vi "RotateDegrees.vi"() -> ()   [LabVIEW 2016]
uses:
  Refname/Motors.ctl
  Refname/Refname to String (Motors).vi
  <vilib>/addons/control/pid/pid.llb/PID (DBL).vi
  <vilib>/addons/control/pid/NI_PID_pid.lvlib
panel:
  in  "Threshold Wheel":dbl format="%#_13g"
  in  "PID Gains Wheel":T1={"proportional gain (Kc)"=1.0, "integral time (Ti, min)"=0.01, "derivative time (Td, min)"=0.0} {"derivative time (Td, min)" format="%.3f"; "integral time (Ti, min)" format="%.3f"; "proportional gain (Kc)" format="%.3f"}
  in  "Threshhold":dbl
  in  "PID gains Swerve":T1={"proportional gain (Kc)"=1.0, "integral time (Ti, min)"=0.01, "derivative time (Td, min)"=0.0} {"derivative time (Td, min)" format="%.3f"; "integral time (Ti, min)" format="%.3f"; "proportional gain (Kc)" format="%.3f"}
  in  "Radians to Turn":dbl format="%#_13g"
  in  "Encoder Position":dbl=22.222 format="%#_13g"
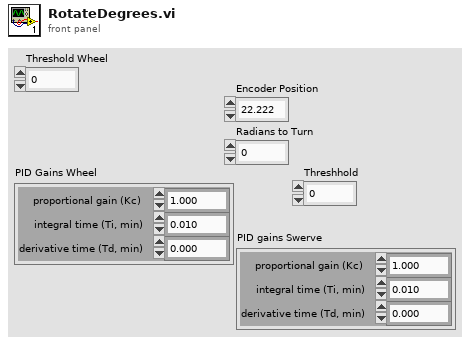
[diagram p1: front panel]
types:
  T1 = cluster{"proportional gain (Kc)":dbl, "integral time (Ti, min)":dbl, "derivative time (Td, min)":dbl}
  T2 = typedef "Motors.ctl" = enum16{"Wheel 1", "Swerve 1", "Wheel 2", "Swerve 2", "Wheel 3", "Swerve 3", "Wheel 4", "Swerve 4"}
  T3 = typedef "WPI_MotorControlDeviceRef.ctl" = cluster{"DeviceStatus":errorcluster, "Type":T4, "PWM":cluster{"PWM Channel":T5, "DeadBand":T6}, "CAN":cluster{"Device Number":u8, "SetOutput VI Ref":variant, "GetOutput VI Ref":variant, "Enable VI Ref":variant, "Disable VI Ref":variant, "Data":variant}, "Invert":bool}
  T4 = typedef "WPI_MotorControlType.ctl" = enum16{"PWM", "CAN"}
  T5 = typedef "FPGA_DIOPWMChannel.ctl" = enum8{"PWM 0", "PWM 1", "PWM 2", "PWM 3", "PWM 4", "PWM 5", "PWM 6", "PWM 7", "PWM 8", "PWM 9", "PWM MXP 0", "PWM MXP 1", "PWM MXP 2", "PWM MXP 3", "PWM MXP 4", "PWM MXP 5", "PWM MXP 6", "PWM MXP 7", "PWM MXP 8", "PWM MXP 9", "Invalid"}
  T6 = typedef "WPI_PWMDeadband.ctl" = cluster{"Name":string, "maxPositivePwm":i32, "minPositivePwm":i32, "centerPwm":i32, "maxNegativePwm":i32, "minNegativePwm":i32, "angularRange":u16}
  T7 = typedef "WPI_CANTalonSRX_GlobalStatus.ctl" = cluster{"Applied Throttle":dbl, "Module Enabled":bool, "CAN Error":errorcluster, "Closed Loop Error":dbl, "Forward Limit Switch Closed":bool, "Reverse Limit Switch Closed":bool, "Sensor Position":dbl, "Sensor Velocity":dbl, "Current":dbl, "Sticky Fault - Over Temp":bool, "Sticky Fault - Under Voltage":bool, "Sticky Fault - Forward Limit":bool, "Sticky Fault - Reverse Limit":bool, "Sticky Fault - Forward Soft Limit":bool, "Sticky Fault - Reverse Soft Limit":bool, "Brake is Enabled":bool, "Encoder Position":dbl, "Encoder Velocity":dbl, "Encoder Index Count":dbl, "Encoder A Pin State":bool, "Encoder B Pin State":bool, "Encoder Index Pin State":bool, "Analog In":dbl, "Analog In Velocity":dbl, "Temperature (C)":dbl, "Battery Voltage":dbl, "Control 5 Is Supported":bool, "Current Profile Slot Select":dbl, "Pos Div 8":bool, "Vel Div 4":bool, "Pulse Width Position":i32, "Pulse Width Velocity":i32, "Pulse Width Rise To Rise (us)":i32, "Pulse Width Rise To Fall (us)":i32, "Mot Prof Active Is Under Run":bool, "Mot Prof Active Has Under Run":bool, "Mot Prof Active Is Last":bool, "Mot Prof Active Velocity Only":bool, "Mot Prof Active Is Valid":bool, "Mot Prof Buffer Is Full":bool, "Mot Prof Active Profile Slot Select":i32, "Mot Prof NextID":i32, "Mot Prof Count":i32, "Mot Prof Active Velocity":dbl, "Mot Prof Active Position":dbl, "Mot Prof Output Enable":i32}
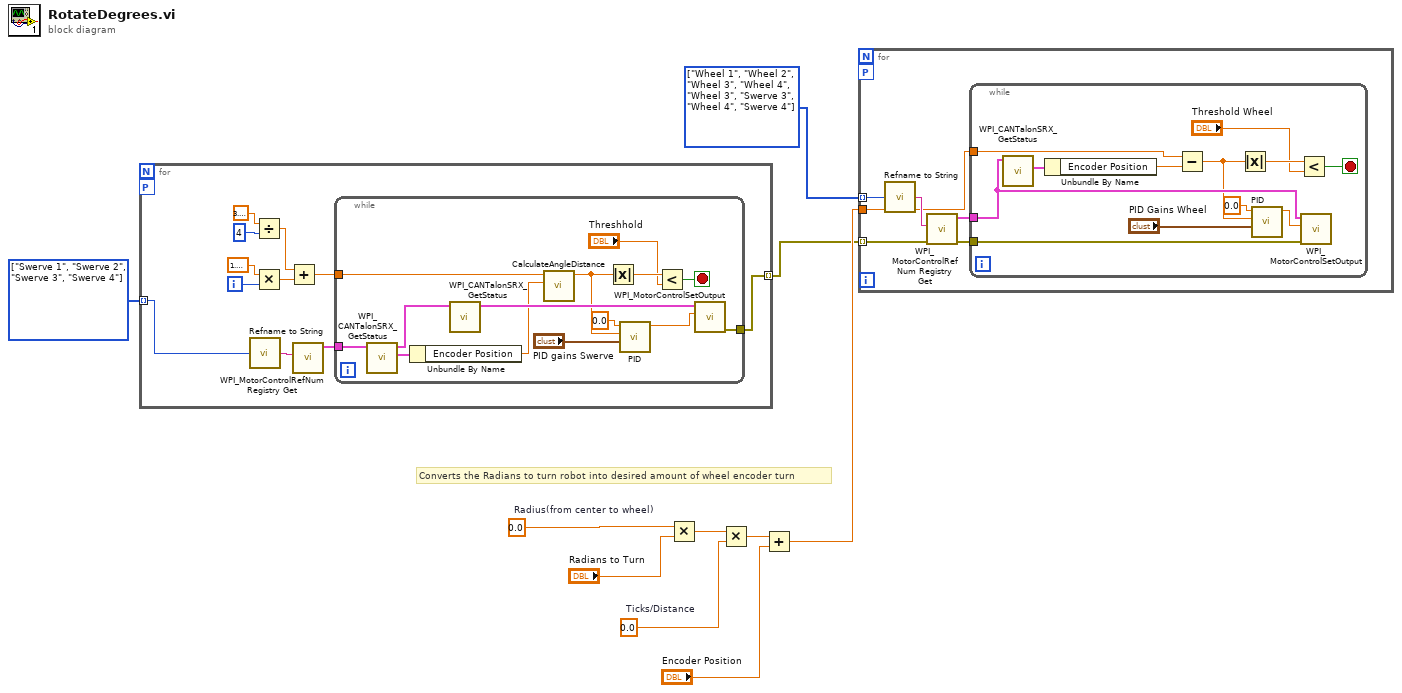
[diagram p0: block diagram]
diagram:
  w2 = T2[] [enum."Swerve 1", enum."Swerve 2", enum."Swerve 3", enum."Swerve 4"] items=["Wheel 1", "Swerve 1", "Wheel 2", "Swerve 2", "Wheel 3", "Swerve 3", "Wheel 4", "Swerve 4"]
  w8 = 0.0  # Ticks/Distance
  w10 = 0.0  # Radius(from center to wheel)
  w4 = T2[] [enum."Wheel 1", enum."Wheel 2", enum."Wheel 3", enum."Wheel 4", enum."Wheel 3", enum."Swerve 3", enum."Wheel 4", enum."Swerve 4"] items=["Wheel 1", "Swerve 1", "Wheel 2", "Swerve 2", "Wheel 3", "Swerve 3", "Wheel 4", "Swerve 4"]
  # "Converts the Radians to turn robot into desired amount of wheel encoder turn"
  n1 = for {
    workers-P: _ -> [_]
    tunnel: w2 -> [w21] mode=indexing
    tunnel: [w13] -> w1 mode=indexing
    i -> [w20]
    n2 = call-poly "Refname to String.vi"("Enum"=w21) -> ("String"=w14:string)
    n3 = Divide(x=3.141592653589793, y=4) -> (x/y=w17:dbl)
    n4 = Multiply(x=1.5707963267948966, y=w20) -> (x*y=w18:dbl)
    n5 = Add(x=w17, y=w18) -> (x+y=w11:dbl)
    n6 = call <vilib>:"WPI_MotorControlRefNum Registry Get.vi"("refnum name"=w14) -> ("MotorControlDevRef"=w12:T3)  [unwired: 9 in, 1 out]
    n7 = while {
      tunnel: [w34] -> w13
      tunnel: w12 -> [w29]
      tunnel: w11 -> [w27]
      stop <- w23 stop-if-true
      n8 = call <vilib>:"WPI_CANTalonSRX_GetStatus.vi"("CAN Talon SRX Ref"=w29) -> ("Talon SRX Status"=w31:T7, "CAN Talon SRX Ref"=w30:T3)  [unwired: 8 in, 1 out]
      n9 = Unbundle By Name(w31) -> ("Encoder Position"=w28:dbl)
      n10 = call <vilib>:"WPI_CANTalonSRX_GetStatus.vi"("CAN Talon SRX Ref"=w30) -> ("CAN Talon SRX Ref"=w35:T3)  [unwired: 8 in, 2 out]
      n11 = call "CalculateAngleDistance.vi"("Current Position"=w28, "Desired Position"=w27) -> ("Distance"=w25:dbl)  [unwired: 9 in]
      n12 = Absolute Value(x=w25) -> (abs(x)=w24:dbl)
      n13 = call-poly <vilib>:"PID.vi"("PID gains"="PID gains Swerve", "process variable"=w25, "setpoint"=0.0) -> ("output"=w26:dbl)  [unwired: 7 in, 1 out]
      n14 = Less?(x=w24, y="Threshhold") -> (x < y?=w23:bool)
      n15 = call <vilib>:"WPI_MotorControlSetOutput.vi"("Output"=w26, "MotorControlDevRef"=w35) -> ("error out"=w34:errorcluster)  [unwired: 7 in, 2 out]
    }
  }
  n16 = Multiply(x=w10, y="Radians to Turn") -> (x*y=w7:dbl)
  n17 = Multiply(x=w7, y=w8) -> (x*y=w5:dbl)
  n18 = Add(x=w5, y="Encoder Position") -> (x+y=w3:dbl)
  n19 = for {
    workers-P: _ -> [_]
    tunnel: w4 -> [w39] mode=indexing
    tunnel: w3 -> [w38]
    tunnel: w1 -> [w36] mode=indexing
    n20 = call-poly "Refname to String.vi"("Enum"=w39) -> ("String"=w41:string)
    n21 = call <vilib>:"WPI_MotorControlRefNum Registry Get.vi"("error in (no error)"=w36, "refnum name"=w41) -> ("error out"=w40:errorcluster, "MotorControlDevRef"=w37:T3)  [unwired: 8 in]
    n22 = while {
      tunnel: w40 -> [w51]
      tunnel: w38 -> [w49]
      tunnel: w37 -> [w52]
      stop <- w42 stop-if-true
      n23 = call <vilib>:"WPI_CANTalonSRX_GetStatus.vi"("CAN Talon SRX Ref"=w52) -> ("Talon SRX Status"=w53:T7)  [unwired: 8 in, 2 out]
      n24 = Unbundle By Name(w53) -> ("Encoder Position"=w48:dbl)
      n25 = Subtract(x=w49, y=w48) -> (x-y=w43:dbl)
      n26 = Absolute Value(x=w43) -> (abs(x)=w45:dbl)
      n27 = call-poly <vilib>:"PID.vi"("PID gains"="PID Gains Wheel", "process variable"=w43, "setpoint"=0.0) -> ("output"=w46:dbl)  [unwired: 7 in, 1 out]
      n28 = Less?(x=w45, y="Threshold Wheel") -> (x < y?=w42:bool)
      n29 = call <vilib>:"WPI_MotorControlSetOutput.vi"("error in (no error)"=w51, "Output"=w46, "MotorControlDevRef"=w52) -> ()  [unwired: 6 in, 3 out]
    }
  }
